vi "filter channels by classification.vi"(10 "allowed classifications":T1[](array[typedef]), 11 "channels in":refnum<class "TBM channel.lvclass">[](array[class])) -> (3 "channels out":refnum<class "TBM channel.lvclass">[](array[class]))   [LabVIEW 2013, in "TBM channel.lvclass"]
doc: "Filters <b>channels in</b> based on the set of allowable classifications"
uses:
  TBM channel.lvclass
  channel classification.ctl
  TBM channel.lvclass/TBM channel.ctl
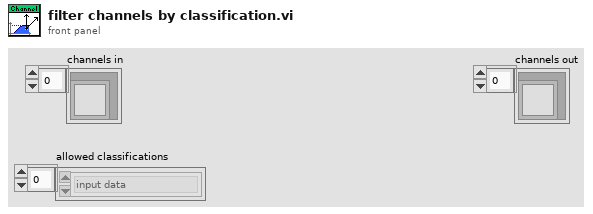
[diagram p1: front panel]
types:
  T1 = typedef "TBM channel.lvclass/channel classification.ctl" = enum16{"input data", "output data", "processing parameter", "processing result"}
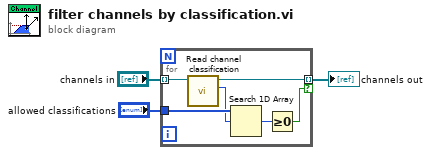
[diagram p0: block diagram]
diagram:
  n1 = for {
    tunnel: "channels in" -> [w6] mode=indexing
    tunnel: "allowed classifications" -> [w9]
    tunnel: [w5] -> w1 mode=indexing if=w7
    n2 = call "Read channel classification.vi"("channel in"=w6) -> ("channel classification"=w4:T1, "channel out"=w5:refnum<class "TBM channel.lvclass">)  [unwired: 8 in, 1 out]
    n3 = Search 1D Array(1D array=w9, element=w4) -> (index of element=w8:i32)  [unwired: 1 in]
    n4 = Greater Or Equal To 0?(x=w8) -> (x >= 0?=w7:bool)
  }
  "channels out" <- w1
